vi "HFRR ADV v07 new software.vi"() -> ()   [LabVIEW 2025] (continued)
                frame 56 {
                  n3116 = local write "S 57"(w4150) -> ()
                }
                frame 57 {
                  n3117 = local write "S 58"(w4151) -> ()
                }
                frame 58 {
                  n3118 = local write "S 59"(w4152) -> ()
                }
                frame 59 {
                  n3119 = local write "S 60"(w4153) -> ()
                }
                frame 60 {
                  n3120 = local write "S 62"(w4154) -> ()
                }
                frame 61 {
                  n3121 = local write "S 63"(w4155) -> ()
                }
                frame 62 {
                  n3122 = local write "S 64"(w4156) -> ()
                }
                frame 63 {
                  n3123 = local write "S 65"(w4157) -> ()
                }
                frame 64 {
                  n3124 = local write "S 66"(w4158) -> ()
                }
                frame 65 {
                  n3125 = local write "S 67"(w4159) -> ()
                }
                frame 66 {
                  n3126 = local write "S 68"(w4160) -> ()
                }
                frame 67 {
                  n3127 = local write "S 69"(w4161) -> ()
                }
                frame 68 {
                  n3128 = local write "S 70"(w4162) -> ()
                }
                frame 69 {
                  n3129 = local write "S 71"(w4163) -> ()
                }
                frame 70 {
                  n3130 = local write "S 72"(w4164) -> ()
                }
                frame 71 {
                  n3131 = local write "S 73"(w4165) -> ()
                }
                frame 72 {
                  n3132 = local write "S 74"(w4166) -> ()
                }
                frame 73 {
                  n3133 = local write "S 75"(w4167) -> ()
                }
                frame 74 {
                  n3134 = local write "S 76"(w4168) -> ()
                }
                frame 75 {
                  n3135 = local write "S 77"(w4169) -> ()
                }
                frame 76 {
                  n3136 = local write "S 78"(w4170) -> ()
                }
                frame 77 {
                  n3137 = local write "S 79"(w4171) -> ()
                }
                frame 79 {
                  n3138 = property on="Sample Temperature ( °C )" class="XYGraph (strict)"("Y Scale.Name Label.Text"=w4172) -> ()  [unwired: 2 in, 2 out]
                }
                frame 80 {
                  n3139 = local write "S 81"(w4173) -> ()
                  n3140 = property on="Humidity ( %RH )" class="XYGraph (strict)"("Y Scale.Name Label.Text"=w4173) -> ()  [unwired: 2 in, 2 out]
                }
                frame 78 {
                  n3141 = property on="Air Temperature  ( °C )" class="XYGraph (strict)"("X Scale.Name Label.Text"=w4174) -> ()  [unwired: 2 in, 2 out]
                  n3142 = property on="Humidity ( %RH )" class="XYGraph (strict)"("X Scale.Name Label.Text"=w4174) -> ()  [unwired: 2 in, 2 out]
                  n3143 = property on="Sample Temperature ( °C )" class="XYGraph (strict)"("X Scale.Name Label.Text"=w4174) -> ()  [unwired: 2 in, 2 out]
                  n3144 = property on="Coefficient Of Friction" class="XYGraph (strict)"("X Scale.Name Label.Text"=w4174) -> ()  [unwired: 2 in, 2 out]
                }
                frame 81 {
                  n3145 = property on="Air Temperature  ( °C )" class="XYGraph (strict)"("Y Scale.Name Label.Text"=w4175) -> ()  [unwired: 2 in, 2 out]
                }
                frame 82 {
                  n3146 = local write "S 84"(w4176) -> ()
                }
                frame 83 {
                  n3147 = local write "S 85"(w4177) -> ()
                }
                frame 84 {
                  n3148 = local write "S 86"(w4178) -> ()
                }
                frame 85 {
                  n3149 = local write "S 87"(w4179) -> ()
                }
                frame 86 {
                  n3150 = local write "S 88"(w4180) -> ()
                }
                frame 87 {
                }
                frame 88 {
                  n3151 = local write "S 90"(w4182) -> ()
                }
                frame 89 {
                  n3152 = local write "S 91"(w4183) -> ()
                }
                frame 90 {
                  n3153 = local write "S 92"(w4184) -> ()
                }
                frame 91 {
                  n3154 = local write "S 93"(w4185) -> ()
                }
                frame 92 {
                  n3155 = local write "S 94"(w4186) -> ()
                }
                frame 93 {
                  n3156 = local write "S 95"(w4187) -> ()
                }
                frame 94 {
                  n3157 = local write "S 96"(w4188) -> ()
                }
                frame 95 {
                  n3158 = local write "S 97"(w4189) -> ()
                }
                frame 96 {
                  n3159 = local write "S 98"(w4190) -> ()
                }
                frame 97 {
                  n3160 = local write "S 99"(w4191) -> ()
                }
                frame 98 {
                  n3161 = local write "S 100"(w4192) -> ()
                }
                frame 99 {
                  n3162 = local write "S 101"(w4193) -> ()
                }
                frame 100 {
                  n3163 = local write "S 102"(w4194) -> ()
                }
                frame 101 {
                  n3164 = local write "S 103"(w4195) -> ()
                }
                frame 102 {
                  n3165 = local write "S 104"(w4196) -> ()
                }
                frame 103 {
                  n3166 = local write "S 105"(w4197) -> ()
                }
                frame 104 {
                  n3167 = local write "S 106"(w4198) -> ()
                }
                frame 105 {
                }
                frame 106 {
                  n3168 = property on="OK Button 17" class="Bool (strict)"("Boolean Text.Text"=w4199) -> ()  [unwired: 2 in, 2 out]
                }
                frame 107 {
                  n3169 = property on="OK Button 16" class="Bool (strict)"("Boolean Text.Text"=w4200) -> ()  [unwired: 2 in, 2 out]
                }
                frame 108 {
                  n3170 = property on="TITTLE" class="Str"("Caption.Text"=w4201) -> ()  [unwired: 2 in, 2 out]
                }
                frame 109 {
                  "String 30" <- w4202
                }
                frame 110 {
                  n3171 = property on="Test Date" class="Str"("Caption.Text"=w4203) -> ()  [unwired: 2 in, 2 out]
                  "String 31" <- w4203
                }
                frame 111 {
                  n3172 = property on="Sample ID" class="Str"("Caption.Text"=w4204) -> ()  [unwired: 2 in, 2 out]
                  "String 32" <- w4204
                }
                frame 112 {
                  n3173 = property on="Tested by" class="Str"("Caption.Text"=w4205) -> ()  [unwired: 2 in, 2 out]
                  "String 33" <- w4205
                }
                frame 113 {
                  n3174 = property on="System Configured Printers 2" class="Arr (strict)"("Caption.Text"=w4206) -> ()  [unwired: 2 in, 2 out]
                }
                frame 114 {
                  n3175 = property on="Selected Printer" class="Str"("Caption.Text"=w4207) -> ()  [unwired: 2 in, 2 out]
                }
                frame 115 {
                  n3176 = property on="Select Printer 3" class="DigNum (strict)"("Caption.Text"=w4208) -> ()  [unwired: 2 in, 2 out]
                }
                frame 116 {
                  n3177 = property on="Print" class="Bool (strict)"("Boolean Text.Text"=w4209) -> ()  [unwired: 2 in, 2 out]
                }
                frame 117 {
                  "String 41" <- w4210
                }
                frame 118 {
                  n3178 = property on="tested by" class="Str"("Caption.Text"=w4211) -> ()  [unwired: 2 in, 2 out]
                }
                frame 119 {
                }
                frame 120 {
                  n3179 = property on="Export" class="Bool (strict)"("Boolean Text.Text"=w4212) -> ()  [unwired: 2 in, 2 out]
                }
                frame 121 {
                  n3180 = property on="TEMP INTERCEPT:" class="DigNum (strict)"("Caption.Text"=w4213) -> ()  [unwired: 2 in, 2 out]
                }
                frame 122 {
                  n3181 = property on="AIR TEMP INTERCEPT:" class="DigNum (strict)"("Caption.Text"=w4214) -> ()  [unwired: 2 in, 2 out]
                }
                frame 123 {
                  n3182 = property on="Select File Type" class="Enum (strict)"("Caption.Text"=w4215) -> ()  [unwired: 2 in, 2 out]
                }
                frame 124 {
                  n3183 = property on="s.NO" class="Str"("Caption.Text"=w4216) -> ()  [unwired: 2 in, 2 out]
                  "String 45" <- w4216
                }
                frame 125 {
                  n3184 = property on="trip1 8" class="Bool (strict)"("Boolean Text.Text"=w4217) -> ()  [unwired: 2 in, 2 out]
                }
                frame 126, Default {
                }
              }
            }
          }
          frame #1 {
            w4225 = TRUE ("Visible")
            n3185 = local read "S 91"() -> (w4242:string)
            n3186 = local read "S 90"() -> (w4241:string)
            n3187 = local read "S 88"() -> (w4240:string)
            n3188 = property on="File Path" class="Path"("Caption.Text"=w4241) -> ()  [unwired: 2 in, 2 out]
            n3189 = property on="SrvM CP" class="Bool (strict)"("Boolean Text.Text"=w4240) -> ()  [unwired: 2 in, 2 out]
            n3190 = local read "S 71"() -> (w4235:string)
            n3191 = local read "S 86"() -> (w4237:string)
            n3192 = local read "S 85"() -> (w4238:string)
            n3193 = local read "S 87"() -> (w4236:string)
            n3194 = local read "S 84"() -> (w4239:string)
            n3195 = local read "S 103"() -> (w4224:string)
            n3196 = local read "S 104"() -> (w4223:string)
            n3197 = property on="ENTER THE NEW PASSWORD" class="Str"("Caption.Text"=w4236) -> ()  [unwired: 2 in, 2 out]
            n3198 = property on="Password" class="Str"("Caption.Text"=w4238) -> ()  [unwired: 2 in, 2 out]
            n3199 = property on="ENTER CURRENT PASSWORD" class="Str"("Caption.Text"=w4237) -> ()  [unwired: 2 in, 2 out]
            n3200 = property on="EDIT" class="Bool (strict)"("Boolean Text.Text"=w4235) -> ()  [unwired: 2 in, 2 out]
            n3201 = property on="SAVE" class="Bool (strict)"("Boolean Text.Text"=w4239) -> ()  [unwired: 2 in, 2 out]
            n3202 = Build Array(w4224, w4223) -> (w4222:string[])
            n3203 = property on="Heater Button" class="Bool (strict)"("Strings [4]"=w4222) -> ()  [unwired: 2 in, 2 out]
            n3204 = property on="CH-HUMIDITY WET" class="DigNum (strict)"("Caption.Size to Text?"=w4225) -> ()  [unwired: 2 in, 2 out]
            n3205 = property on="CH-HUMIDITY DRY" class="DigNum (strict)"("Caption.Size to Text?"=w4225) -> ()  [unwired: 2 in, 2 out]
            n3206 = property on="CH-POWER -" class="DigNum (strict)"("Caption.Size to Text?"=w4225) -> ()  [unwired: 2 in, 2 out]
            n3207 = property on="CH-HEATER" class="DigNum (strict)"("Caption.Size to Text?"=w4225) -> ()  [unwired: 2 in, 2 out]
            n3208 = property on="CH-POWER +" class="DigNum (strict)"("Caption.Size to Text?"=w4225) -> ()  [unwired: 2 in, 2 out]
            n3209 = local read "S 92"() -> (w4234:string)
            n3210 = local read "S 93"() -> (w4233:string)
            n3211 = local read "S 105"() -> (w4220:string)
            n3212 = local read "S 106"() -> (w4219:string)
            n3213 = Build Array(w4234, w4233) -> ()  [unwired: 1 out]
            n3214 = Build Array(w4220, w4219) -> (w4221:string[])
            n3215 = local read "S 95"() -> (w4231:string)
            n3216 = local read "S 94"() -> (w4232:string)
            n3217 = local read "bs"() -> (w4247:string)
            n3218 = local read "as"() -> (w4248:string)
            n3219 = property on="Humidity" class="Bool (strict)"("Strings [4]"=w4221) -> ()  [unwired: 2 in, 2 out]
            n3220 = Concatenate Strings(w4247, "\r", w4248) -> ()  [unwired: 1 out]
            n3221 = property on="STROKE GAIN :" class="DigNum (strict)"("Caption.Text"=w4231) -> ()  [unwired: 2 in, 2 out]
            n3222 = property on="DISPLACEMENT :" class="DigNum (strict)"("Caption.Text"=w4232) -> ()  [unwired: 2 in, 2 out]
            n3223 = property on="Rh After" class="DigNum (strict)"("Caption.Size to Text?"=TRUE ("Caption.Size to Text")) -> ()  [unwired: 2 in, 2 out]
            n3224 = local read "S 48"() -> (w4271:string)
            n3225 = local read "S 50"() -> (w4269:string)
            n3226 = local read "S 51"() -> (w4268:string)
            n3227 = local read "S 49"() -> (w4270:string)
            n3228 = local read "S 52"() -> (w4267:string)
            n3229 = local read "as"() -> (w4252:string)
            n3230 = local read "bs"() -> (w4253:string)
            n3231 = local read "S 56"() -> (w4266:string)
            n3232 = local read "S 57"() -> (w4265:string)
            n3233 = local read "S 58"() -> (w4264:string)
            n3234 = local read "S 59"() -> (w4263:string)
            n3235 = property on="OPEN" class="Bool (strict)"("Boolean Text.Text"=w4267) -> ()  [unwired: 2 in, 2 out]
            n3236 = property on="OPEN 1" class="Bool (strict)"("Boolean Text.Text"=w4271) -> ()  [unwired: 2 in, 2 out]
            n3237 = property on="OPEN 2" class="Bool (strict)"("Boolean Text.Text"=w4270) -> ()  [unwired: 2 in, 2 out]
            n3238 = property on="OPEN 3" class="Bool (strict)"("Boolean Text.Text"=w4269) -> ()  [unwired: 2 in, 2 out]
            n3239 = property on="OPEN 4" class="Bool (strict)"("Boolean Text.Text"=w4268) -> ()  [unwired: 2 in, 2 out]
            n3240 = Concatenate Strings(w4253, "\r", w4252) -> ()  [unwired: 1 out]
            n3241 = local read "S 102"() -> (w4226:string)
            n3242 = property on="КОФ1" class="DigNum (strict)"("Caption.Text"=w4266) -> ()  [unwired: 2 in, 2 out]
            n3243 = local read "S 98"() -> (w4230:string)
            n3244 = local read "S 99"() -> (w4229:string)
            n3245 = local read "S 100"() -> (w4228:string)
            n3246 = local read "S 101"() -> (w4227:string)
            n3247 = property on="КОФ2" class="DigNum (strict)"("Caption.Text"=w4265) -> ()  [unwired: 2 in, 2 out]
            n3248 = property on="КОФ3" class="DigNum (strict)"("Caption.Text"=w4264) -> ()  [unwired: 2 in, 2 out]
            n3249 = property on="КОФ4" class="DigNum (strict)"("Caption.Text"=w4263) -> ()  [unwired: 2 in, 2 out]
            n3250 = local read "bs"() -> (w4251:string)
            n3251 = local read "as"() -> (w4250:string)
            n3252 = property on="CH-POWER +" class="DigNum (strict)"("Caption.Text"=w4230) -> ()  [unwired: 2 in, 2 out]
            n3253 = property on="CH-POWER -" class="DigNum (strict)"("Caption.Text"=w4229) -> ()  [unwired: 2 in, 2 out]
            n3254 = property on="CH-HEATER" class="DigNum (strict)"("Caption.Text"=w4228) -> ()  [unwired: 2 in, 2 out]
            n3255 = property on="CH-HUMIDITY DRY" class="DigNum (strict)"("Caption.Text"=w4227) -> ()  [unwired: 2 in, 2 out]
            n3256 = property on="CH-HUMIDITY WET" class="DigNum (strict)"("Caption.Text"=w4226) -> ()  [unwired: 2 in, 2 out]
            n3257 = local read "S 60"() -> (w4262:string)
            n3258 = local read "S 54"() -> (w4272:string)
            n3259 = Concatenate Strings(w4251, "\r", w4250) -> ()  [unwired: 1 out]
            n3260 = Concatenate Strings(w4272, w4262) -> ()  [unwired: 1 out]
            n3261 = local read "S 77"() -> (→"String 43":string)
            n3262 = local read "S 76"() -> (w4245:string)
            n3263 = local read "S 78"() -> (w4244:string)
            n3264 = local read "S 71"() -> (w4256:string)
            n3265 = local read "S 66"() -> (w4261:string)
            n3266 = local read "S 67"() -> (w4260:string)
            n3267 = local read "S 68"() -> (w4259:string)
            n3268 = local read "S 69"() -> (w4258:string)
            n3269 = local read "S 70"() -> (w4257:string)
            n3270 = property on="AIR TEMP" class="DigNum (strict)"("Caption.Text"=w4244) -> ()  [unwired: 2 in, 2 out]
            n3271 = property on="Set Strk" class="DigNum (strict)"("Caption.Text"=w4245) -> ()  [unwired: 2 in, 2 out]
            n3272 = property on="FRIC. FORCE :" class="DigNum (strict)"("Caption.Text"=w4261) -> ()  [unwired: 2 in, 2 out]
            n3273 = property on="TEMPERATURE :" class="DigNum (strict)"("Caption.Text"=w4260) -> ()  [unwired: 2 in, 2 out]
            n3274 = property on="SPEED OUT:" class="DigNum (strict)"("Caption.Text"=w4259) -> ()  [unwired: 2 in, 2 out]
            n3275 = property on="AIR TEMPERATURE :" class="DigNum (strict)"("Caption.Text"=w4258) -> ()  [unwired: 2 in, 2 out]
            n3276 = property on="HUMIDITY:" class="DigNum (strict)"("Caption.Text"=w4257) -> ()  [unwired: 2 in, 2 out]
            n3277 = property on="EDIT" class="Bool (strict)"("Boolean Text.Text"=w4256) -> ()  [unwired: 2 in, 2 out]
            n3278 = local read "S 79"() -> (w4243:string)
          }
          frame #2 {
          }
        }
        n3279 = local write "Lan flag"(10.0 ("Lan flag")) -> ()
      }
      frame Enabled {
      }
    }
    n3280 = Wait (ms)(milliseconds to wait=u32 2000) -> ()  [unwired: 1 out]
    n3281 = local read "Quit"() -> (w4046:bool)
  }
  n3282 = disable-structure shown="Disabled" {
    frame Disabled {
      n3283 = while {
        tunnel: [w4274] -> _
        i -> [w4274]
        stop <- w4273 continue-if-true
        n3284 = Wait (ms)(milliseconds to wait=u32 50) -> ()  [unwired: 1 out]
        n3285 = stacked-sequence {
          frame #0 {
            # "Controls Text color"
            # "Controls BG color"
            n3286 = property on="FILE" class="Str"("Text.Text Colors:Text Color"="SC  Text") -> ()  [unwired: 2 in, 2 out]
            n3287 = property on="Fuel Discription :" class="Str"("Text.Text Colors:Text Color"="SC  Text") -> ()  [unwired: 2 in, 2 out]
            n3288 = property on="tested by" class="Str"("Text.Text Colors:Text Color"="SC  Text") -> ()  [unwired: 2 in, 2 out]
            n3289 = property on="Remarks :" class="Str"("Text.Text Colors:Text Color"="SC  Text") -> ()  [unwired: 2 in, 2 out]
            n3290 = property class="DigNum (strict)"("Numeric Text.Text Colors:BG Color"="NC BG") -> ()  [unwired: 2 in, 2 out]
            n3291 = property class="DigNum (strict)"("Numeric Text.Text Colors:BG Color"="NC BG") -> ()  [unwired: 2 in, 2 out]
            n3292 = property class="DigNum (strict)"("Numeric Text.Text Colors:BG Color"="NC BG") -> ()  [unwired: 2 in, 2 out]
            n3293 = property class="DigNum (strict)"("Numeric Text.Text Colors:BG Color"="NC BG") -> ()  [unwired: 2 in, 2 out]
            n3294 = property class="DigNum (strict)"("Numeric Text.Text Colors:BG Color"="NC BG") -> ()  [unwired: 2 in, 2 out]
            n3295 = property class="DigNum (strict)"("Numeric Text.Text Colors:BG Color"="NC BG") -> ()  [unwired: 2 in, 2 out]
            n3296 = property class="DigNum (strict)"("Numeric Text.Text Colors:BG Color"="NC BG") -> ()  [unwired: 2 in, 2 out]
            n3297 = property class="DigNum (strict)"("Numeric Text.Text Colors:BG Color"="NC BG") -> ()  [unwired: 2 in, 2 out]
            n3298 = property class="DigNum (strict)"("Numeric Text.Text Colors:BG Color"="NC BG") -> ()  [unwired: 2 in, 2 out]
            n3299 = property class="DigNum (strict)"("Numeric Text.Text Colors:BG Color"="NC BG") -> ()  [unwired: 2 in, 2 out]
            n3300 = property class="DigNum (strict)"("Numeric Text.Text Colors:BG Color"="NC BG") -> ()  [unwired: 2 in, 2 out]
            n3301 = property class="DigNum (strict)"("Numeric Text.Text Colors:BG Color"="NC BG") -> ()  [unwired: 2 in, 2 out]
            n3302 = property on="FILE" class="Str"("Text.Text Colors:BG Color"="SC BG 3") -> ()  [unwired: 2 in, 2 out]
            n3303 = property on="Fuel Discription :" class="Str"("Text.Text Colors:BG Color"="SC BG 3") -> ()  [unwired: 2 in, 2 out]
            n3304 = property on="tested by" class="Str"("Text.Text Colors:BG Color"="SC BG 3") -> ()  [unwired: 2 in, 2 out]
            n3305 = property on="Remarks :" class="Str"("Text.Text Colors:BG Color"="SC BG 3") -> ()  [unwired: 2 in, 2 out]
            n3306 = property class="DigNum (strict)"("Numeric Text.Text Colors:Text Color"="NC Text") -> ()  [unwired: 2 in, 2 out]
            n3307 = property class="DigNum (strict)"("Numeric Text.Text Colors:Text Color"="NC Text") -> ()  [unwired: 2 in, 2 out]
            n3308 = property class="DigNum (strict)"("Numeric Text.Text Colors:Text Color"="NC Text") -> ()  [unwired: 2 in, 2 out]
            n3309 = property class="DigNum (strict)"("Numeric Text.Text Colors:Text Color"="NC Text") -> ()  [unwired: 2 in, 2 out]
            n3310 = property class="DigNum (strict)"("Numeric Text.Text Colors:Text Color"="NC Text") -> ()  [unwired: 2 in, 2 out]
            n3311 = property class="DigNum (strict)"("Numeric Text.Text Colors:Text Color"="NC Text") -> ()  [unwired: 2 in, 2 out]
            n3312 = property class="DigNum (strict)"("Numeric Text.Text Colors:Text Color"="NC Text") -> ()  [unwired: 2 in, 2 out]
            n3313 = property class="DigNum (strict)"("Numeric Text.Text Colors:Text Color"="NC Text") -> ()  [unwired: 2 in, 2 out]
            n3314 = property class="DigNum (strict)"("Numeric Text.Text Colors:Text Color"="NC Text") -> ()  [unwired: 2 in, 2 out]
            n3315 = property class="DigNum (strict)"("Numeric Text.Text Colors:Text Color"="NC Text") -> ()  [unwired: 2 in, 2 out]
            n3316 = property class="DigNum (strict)"("Numeric Text.Text Colors:Text Color"="NC Text") -> ()  [unwired: 2 in, 2 out]
            n3317 = property class="DigNum (strict)"("Numeric Text.Text Colors:Text Color"="NC Text") -> ()  [unwired: 2 in, 2 out]
            n3318 = property class="DigNum (strict)"("Numeric Text.Text Colors:Text Color"="NI Text  2") -> ()  [unwired: 2 in, 2 out]
            n3319 = property class="DigNum (strict)"("Numeric Text.Text Colors:Text Color"="NI Text  2") -> ()  [unwired: 2 in, 2 out]
            n3320 = property class="DigNum (strict)"("Numeric Text.Text Colors:Text Color"="NI Text  2") -> ()  [unwired: 2 in, 2 out]
            n3321 = property class="DigNum (strict)"("Numeric Text.Text Colors:Text Color"="NI Text  2") -> ()  [unwired: 2 in, 2 out]
            n3322 = property class="DigNum (strict)"("Numeric Text.Text Colors:Text Color"="NI Text  2") -> ()  [unwired: 2 in, 2 out]
            n3323 = property class="DigNum (strict)"("Numeric Text.Text Colors:Text Color"="NI Text  2") -> ()  [unwired: 2 in, 2 out]
            n3324 = property class="DigNum (strict)"("Numeric Text.Text Colors:Text Color"="NI Text  2") -> ()  [unwired: 2 in, 2 out]
            n3325 = property class="DigNum (strict)"("Numeric Text.Text Colors:Text Color"="NI Text  2") -> ()  [unwired: 2 in, 2 out]
            n3326 = property class="DigNum (strict)"("Numeric Text.Text Colors:Text Color"="NI Text  2") -> ()  [unwired: 2 in, 2 out]
            n3327 = property class="DigNum (strict)"("Numeric Text.Text Colors:Text Color"="NI Text  2") -> ()  [unwired: 2 in, 2 out]
            n3328 = property class="DigNum (strict)"("Numeric Text.Text Colors:Text Color"="NI Text  2") -> ()  [unwired: 2 in, 2 out]
            n3329 = property class="DigNum (strict)"("Numeric Text.Text Colors:Text Color"="NI Text  2") -> ()  [unwired: 2 in, 2 out]
            n3330 = property class="DigNum (strict)"("Numeric Text.Text Colors:Text Color"="NI Text  2") -> ()  [unwired: 2 in, 2 out]
            n3331 = property class="DigNum (strict)"("Numeric Text.Text Colors:Text Color"="NI Text  2") -> ()  [unwired: 2 in, 2 out]
            n3332 = property class="DigNum (strict)"("Numeric Text.Text Colors:Text Color"="NI Text  2") -> ()  [unwired: 2 in, 2 out]
            n3333 = property on="Coefficient Of Friction" class="XYGraph (strict)"("Plot Area:Colors:FG Color"="GFG  2", "Plot Area:Colors:BG Color"="GBG   2") -> ()  [unwired: 2 in, 2 out]
            n3334 = property on="Humidity ( %RH )" class="XYGraph (strict)"("Plot Area:Colors:FG Color"="GFG  2", "Plot Area:Colors:BG Color"="GBG   2") -> ()  [unwired: 2 in, 2 out]
            n3335 = property on="Air Temperature  ( °C )" class="XYGraph (strict)"("Plot Area:Colors:FG Color"="GFG  2", "Plot Area:Colors:BG Color"="GBG   2") -> ()  [unwired: 2 in, 2 out]
            n3336 = property on="Sample Temperature ( °C )" class="XYGraph (strict)"("Plot Area:Colors:FG Color"="GFG  2", "Plot Area:Colors:BG Color"="GBG   2") -> ()  [unwired: 2 in, 2 out]
            n3337 = property class="DigNum (strict)"("Numeric Text.Text Colors:BG Color"="NI BG 2") -> ()  [unwired: 2 in, 2 out]
            n3338 = property class="DigNum (strict)"("Numeric Text.Text Colors:BG Color"="NI BG 2") -> ()  [unwired: 2 in, 2 out]
            n3339 = property class="DigNum (strict)"("Numeric Text.Text Colors:BG Color"="NI BG 2") -> ()  [unwired: 2 in, 2 out]
            n3340 = property class="DigNum (strict)"("Numeric Text.Text Colors:BG Color"="NI BG 2") -> ()  [unwired: 2 in, 2 out]
            n3341 = property class="DigNum (strict)"("Numeric Text.Text Colors:BG Color"="NI BG 2") -> ()  [unwired: 2 in, 2 out]
            n3342 = property class="DigNum (strict)"("Numeric Text.Text Colors:BG Color"="NI BG 2") -> ()  [unwired: 2 in, 2 out]
            n3343 = property class="DigNum (strict)"("Numeric Text.Text Colors:BG Color"="NI BG 2") -> ()  [unwired: 2 in, 2 out]
            n3344 = property class="DigNum (strict)"("Numeric Text.Text Colors:BG Color"="NI BG 2") -> ()  [unwired: 2 in, 2 out]
            n3345 = property class="DigNum (strict)"("Numeric Text.Text Colors:BG Color"="NI BG 2") -> ()  [unwired: 2 in, 2 out]
            n3346 = property class="DigNum (strict)"("Numeric Text.Text Colors:BG Color"="NI BG 2") -> ()  [unwired: 2 in, 2 out]
            n3347 = property class="DigNum (strict)"("Numeric Text.Text Colors:BG Color"="NI BG 2") -> ()  [unwired: 2 in, 2 out]
            n3348 = property class="DigNum (strict)"("Numeric Text.Text Colors:BG Color"="NI BG 2") -> ()  [unwired: 2 in, 2 out]
            n3349 = property class="DigNum (strict)"("Numeric Text.Text Colors:BG Color"="NI BG 2") -> ()  [unwired: 2 in, 2 out]
            n3350 = property class="DigNum (strict)"("Numeric Text.Text Colors:BG Color"="NI BG 2") -> ()  [unwired: 2 in, 2 out]
            n3351 = property class="DigNum (strict)"("Numeric Text.Text Colors:BG Color"="NI BG 2") -> ()  [unwired: 2 in, 2 out]
            n3352 = property class="Bool"("Colors [4]"="Boolean BC T & BG") -> ()  [unwired: 2 in, 2 out]
            n3353 = property on="Save & Continue" class="Bool (strict)"("Colors [4]"="Boolean BC T & BG") -> ()  [unwired: 2 in, 2 out]
            n3354 = property on="Heater Button" class="Bool (strict)"("Colors [4]"="Boolean BC T & BG") -> ()  [unwired: 2 in, 2 out]
            n3355 = property class="Bool"("Colors [4]"="Boolean BC T & BG") -> ()  [unwired: 2 in, 2 out]
            n3356 = property on="Humidity" class="Bool (strict)"("Colors [4]"="Boolean BC T & BG") -> ()  [unwired: 2 in, 2 out]
            n3357 = property class="Bool (strict)"("Colors [4]"="Boolean BC T & BG") -> ()  [unwired: 2 in, 2 out]
            n3358 = property on="RUN" class="Bool (strict)"("Colors [4]"="Boolean BC T & BG") -> ()  [unwired: 2 in, 2 out]
            n3359 = property on="trip1 8" class="Bool (strict)"("Colors [4]"="Boolean BC T & BG") -> ()  [unwired: 2 in, 2 out]
            n3360 = property class="Bool"("Colors [4]"="Boolean BC T & BG") -> ()  [unwired: 2 in, 2 out]
            n3361 = property class="Bool (strict)"("Colors [4]"="Boolean BC T & BG") -> ()  [unwired: 2 in, 2 out]
            n3362 = property on="OPEN 1" class="Bool (strict)"("Colors [4]"="Boolean BC T & BG 2") -> ()  [unwired: 2 in, 2 out]
            n3363 = property on="OPEN 2" class="Bool (strict)"("Colors [4]"="Boolean BC T & BG 2") -> ()  [unwired: 2 in, 2 out]
            n3364 = property on="OPEN 3" class="Bool (strict)"("Colors [4]"="Boolean BC T & BG 2") -> ()  [unwired: 2 in, 2 out]
            n3365 = property on="OPEN 4" class="Bool (strict)"("Colors [4]"="Boolean BC T & BG 2") -> ()  [unwired: 2 in, 2 out]
            n3366 = property on="OPEN" class="Bool (strict)"("Colors [4]"="Boolean BC T & BG 2") -> ()  [unwired: 2 in, 2 out]
            n3367 = property on="rstv2" class="Bool"("Colors [4]"="Boolean BC T & BG 2") -> ()  [unwired: 2 in, 2 out]
            n3368 = property on="RST CP" class="Bool"("Colors [4]"="Boolean BC T & BG 2") -> ()  [unwired: 2 in, 2 out]
            n3369 = property on="RSTV1 3" class="Bool"("Colors [4]"="Boolean BC T & BG 2") -> ()  [unwired: 2 in, 2 out]
            n3370 = property on="RSTV1 2" class="Bool"("Colors [4]"="Boolean BC T & BG 2") -> ()  [unwired: 2 in, 2 out]
          }
          frame #1 {
          }
        }
        n3371 = local read "Quit"() -> (w4273:bool)
      }
    }
    frame Enabled {
    }
  }
  n3372 = while {
    shift-right: [w4291] -> _
    shift-left: _ -> [w4292]
    shift-right: [w4289] -> _
    shift-left: T16 {"Read Heave and Surge"="", "Bytes at Heave Port"=0.0, "Heave and Surge COM Port:"="COM9", "Com Port 2"="COM7", "Residual Due"="", "Heave COM Status 2"=TRUE, "Heave COM Status"=TRUE, "Port 2"=TRUE, "Sway PPR"=6400.0, "Surge PPR"=6400.0, "Heave PPR"=6400.0, "Sway Pitch"=2.0, "Surge Pitch"=3.0, "Heave Pitch"=4.0, "Sway Pulses/mm"=320.0, "Surge Pulses/mm"=1600.0, "Heave Pulses/mm"=1600.0, "inner loop"=0.0, "Read Heave and Surge 2"="", "String 36"="", "Write S"=FALSE, "WriteCC1"=[""], "Heave COM Loop"=0, "LastCom"="", "EXIT"=FALSE, "Error Heave"={"status"=TRUE, "code"=-1073807343, "source"=""}} -> [w4288]
    shift-right: [w4286] -> _
    shift-left: enum16{"init", "MAIN", "Panel Close"}."init" -> [w4287]
    stop <- w4290 stop-if-true
    n3373 = case shown="\"MAIN\"" w4287 {
      tunnel: w4292 -> [w4306 w4321 w4391 w4393]
      tunnel: [w4300 w4339 w4391 w4393] -> w4291
      tunnel: [_ _ TRUE _] -> w4290
      tunnel: [w4296 w4336 w4389 w4392] -> w4289
      tunnel: w4288 -> [w4303 w4320 w4389 w4392]
      tunnel: [enum16{"init", "MAIN", "Panel Close"}."MAIN" w4314 _ _] -> w4286
      frame "init" {
        n3374 = Bundle By Name(cluster=w4303, "Heave and Surge COM Port:"="C3 :") -> (w4302:T16)
        n3375 = call "Instrument fgv.vi"("Enum"=T28."INIT", "error in (no error) 2"=w4306, "INPUT"=w4302) -> ("error"=w4304:errorcluster, "output"=w4299:T16)  [unwired: 6 in, 1 out]
        n3376 = case shown="No Error" w4304 {
          selector: w4304 -> [w4308 _]
          tunnel: [w4308 w4312] -> w4300
          tunnel: w4299 -> [w4307 w4310]
          tunnel: [w4307 w4309] -> w4297
          frame No Error {
          }
          frame Error {
            n3377 = call "Instrument fgv.vi"("Enum"=T28."ERROR INIT", "INPUT"=w4310) -> ("error"=w4313:errorcluster, "output"=w4309:T16)  [unwired: 7 in, 1 out]
            n3378 = call <vilib>:"Clear Errors.vi"("error in (no error)"=w4313) -> ("error out"=w4312:errorcluster)  [unwired: 5 in, 1 out]
          }
        }
        n3379 = local read "LastCom"() -> (w4295:string)
        n3380 = Unbundle By Name(w4297) -> ("Heave COM Status 2"=→"COM Status" →"Instrument Status":bool, "Error Heave"=→"Error":errorcluster)  [unwired: 1 out]
        n3381 = Bundle By Name(cluster=w4297, "LastCom"=w4295) -> (w4296:T16)
      }
      frame "MAIN" {
        n3382 = Unbundle By Name(w4320) -> ("Com Port 2"=w4341:refnum<visa-resource-name>)
        n3383 = local write "Com Port 4"(w4341) -> ()
        n3384 = local read "C3 :"() -> (w4318:refnum<visa-resource-name>)
        n3385 = Divide(x="Heave PPR", y="Heave Pitch") -> (x/y=→"Heave Pulses/mm":dbl)
        n3386 = Bundle By Name(cluster=w4320, "Heave and Surge COM Port:"=w4318) -> (w4319:T16)
        n3387 = Equal?(x=w4341, y=w4318) -> (x = y?=w4340:bool)
        n3388 = Divide(x="Sway PPR", y="Sway Pitch") -> (x/y=→"Sway Pulses/mm":dbl)
        n3389 = case shown="False" w4340 {
          tunnel: [w4345 w4362] -> w4339
          tunnel: w4321 -> [w4346 w4368]
          tunnel: w4319 -> [w4344 w4366]
          tunnel: [w4343 w4361] -> w4336
          frame False {
            n3390 = call <vilib>:"Clear Errors.vi"("error in (no error)"=w4346) -> ("error out"=w4342:errorcluster)  [unwired: 5 in, 1 out]
            n3391 = call "Instrument fgv.vi"("Enum"=T28."ERROR INIT", "error in (no error) 2"=w4342, "INPUT"=w4344) -> ("error"=w4348:errorcluster, "output"=w4343:T16)  [unwired: 6 in, 1 out]
            n3392 = call <vilib>:"Clear Errors.vi"("error in (no error)"=w4348) -> ("error out"=w4345:errorcluster)  [unwired: 5 in, 1 out]
          }
          frame True {
            n3393 = call "Instrument fgv.vi"("Enum"=T28."READ", "error in (no error) 2"=w4368, "INPUT"=w4366) -> ("error"=w4367:errorcluster, "output"=w4358:T16)  [unwired: 6 in, 1 out]
            n3394 = Bundle By Name(cluster=w4358, "String 36"="String 11") -> (w4357:T16)
            n3395 = case shown="True" "Write S" {
              selector: "Write S" -> [_ w4388]
              tunnel: w4367 -> [w4381 w4387]
              tunnel: [w4381 w4386] -> w4354
              tunnel: w4357 -> [w4380 w4383]
              tunnel: [w4380 w4382] -> w4353
              frame False {
              }
              frame True {
                n3396 = Not(x=w4388) -> (.not. x?=w4384:bool)
                n3397 = local write "Write S"(w4384) -> ()
                n3398 = call "Instrument fgv.vi"("Enum"=T28."MANUAL WRITE", "error in (no error) 2"=w4387, "INPUT"=w4383) -> ("error"=w4386:errorcluster, "output"=w4382:T16)  [unwired: 6 in, 1 out]
              }
            }
            n3399 = Array Size(array="WriteHumidity") -> (size(s)=w4351:i32)
            n3400 = Greater Than 0?(x=w4351) -> (x > 0?=w4349:bool)
            n3401 = call "Instrument fgv.vi"("Enum"=T28."WRITE", "error in (no error) 2"=w4354, "WriteCC1"="WriteHumidity", "INPUT"=w4353) -> ("error"=w4364:errorcluster, "WriteCC1 2"=w4352:string[], "output"=w4363:T16)  [unwired: 5 in]
            n3402 = case shown="True" w4349 {
              tunnel: w4352 -> [_ w4370]
              frame False {
              }
              frame True {
                n3403 = local write "WriteHumidity"(w4370) -> ()
              }
            }
            n3404 = case shown="Error" w4364 {
              selector: w4364 -> [w4371 w4374]
              tunnel: w4363 -> [w4372 w4379]
              tunnel: [w4372 w4378] -> w4361
              tunnel: [w4371 w4376] -> w4362
              frame No Error {
              }
              frame Error {
                n3405 = call <vilib>:"Clear Errors.vi"("error in (no error)"=w4374) -> ("error out"=w4373:errorcluster)  [unwired: 5 in, 1 out]
                n3406 = call "Instrument fgv.vi"("Enum"=T28."ERROR INIT", "error in (no error) 2"=w4373, "INPUT"=w4379) -> ("error"=w4377:errorcluster, "output"=w4378:T16)  [unwired: 6 in, 1 out]
                n3407 = call <vilib>:"Clear Errors.vi"("error in (no error)"=w4377) -> ("error out"=w4376:errorcluster)  [unwired: 5 in, 1 out]
              }
            }
            n3408 = Unbundle By Name(w4361) -> ("LastCom"=→"LastCom":string, "Read Heave and Surge"=→"Read Humidity":string)
          }
        }
        n3409 = Divide(x="Surge PPR", y="Surge Pitch") -> (x/y=→"Surge Pulses/mm":dbl)
        n3410 = Unbundle By Name(w4336) -> ("Heave COM Status 2"=w4338:bool, "Heave COM Status"=w4337:bool, "Error Heave"=w4334:errorcluster, "Bytes at Heave Port"=→"Bytes at Humidity Port":dbl)
        n3411 = Unbundle By Name(w4334) -> ("status"=→"Humidity Port":bool)
        n3412 = Not(x=w4337) -> (.not. x?=w4322:bool)
        n3413 = local write "Error"(w4334) -> ()
        n3414 = Not(x=w4338) -> (.not. x?=w4323:bool)
        n3415 = local write "Instrument Status"(w4322) -> ()
        n3416 = local write "COM Status"(w4323) -> ()
        n3417 = local read "Quit"() -> (w4315:bool)
        n3418 = Select(t=enum16{"init", "MAIN", "Panel Close"}."Panel Close", s=w4315, f=enum16{"init", "MAIN", "Panel Close"}."MAIN") -> (s? t:f=w4314:enum16{"init", "MAIN", "Panel Close"})
      }
      frame "Panel Close" {
      }
      frame Default {
      }
    }
  }
  n3419 = while {
    stop <- w4419 stop-if-true
    n3420 = local read "Read Humidity"() -> (w4400:string)
    n3421 = call <vilib>:"High Resolution Polling Wait.vi"("seconds to wait"=0.1) -> ()  [unwired: 10 in, 1 out]
    n3422 = Spreadsheet String To Array(delimiter (Tab)=",", format string="", spreadsheet string=w4400, array type (2D Dbl)=string[] []) -> (array=w4414:string[])
    n3423 = for {
      tunnel: w4414 -> [w4424] mode=indexing
      tunnel: string[] ["STATE;", "SET;", "RH;", "T;", "AMB_RH;", "AMB_T;", "PUMP;", "FAN_IN;", "FAN_OUT;", "DEHUM;", "CURRENT;", "STALL;"] -> [w4423] mode=indexing
      tunnel: [w4422] -> w4413 mode=indexing
      n3424 = Match Pattern(string=w4424, regular expression=w4423) -> (after substring=w4422:string)  [unwired: 1 in, 3 out]
    }
    n3425 = Index Array(array=w4413) -> (element #1=→"STATE :":string, element #2=→"SET :":string, element #3=w4402:string, element #4=→"T :":string, element #5=w4399:string, element #6=→"AMB_T :":string, element #7=→"PUMP :":string, element #8=→"FAN_IN :":string, element #9=→"FAN_OUT :":string, element #10=→"DEHUM :":string, element #11=→"CURRENT :":string, element #12=→"STALL :":string)  [unwired: 12 in]
    "RH :" <- w4402
    "AMB_RH :" <- w4399
    n3426 = Fract/Exp String To Number(string=w4402) -> (number=w4394:dbl)  [unwired: 3 in, 1 out]
    n3427 = Fract/Exp String To Number(string=w4399) -> (number=w4398:dbl)  [unwired: 3 in, 1 out]
    n3428 = local write "Ambient Humidity :"(w4398) -> ()
    n3429 = Equal?(x=w4394, y=0.0) -> (x = y?=w4396:bool)
    n3430 = case shown="True" w4396 {
      tunnel: [w4420 w4421] -> w4395
      tunnel: w4394 -> [w4420 _]
      frame False {
        (unwired) 0.0
        "Humidity temp" <- w4420
      }
      frame True {
        n3431 = local read "Humidity temp"() -> (w4421:dbl)
      }
    }
    "RH Numeric:" <- w4395
    n3432 = local read "Quit"() -> (w4419:bool)
  }
  n3433 = disable-structure shown="Disabled" {
    frame Disabled {
      n3434 = while {
        tunnel: [w4658] -> _
        i -> [w4658]
        stop <- w4655 stop-if-true
        n3435 = local read "powstat"() -> (w4656:bool)
        n3436 = case shown="True" w4656 {
          frame False {
          }
          frame True {
            n3437 = local read "RUN"() -> (w4659:bool)
            n3438 = case shown="True" w4659 {
              frame False {
                w4689 = 65.0 ("y")
                n3439 = local read "Set Hz"() -> (w4717:dbl)
                n3440 = local read "NORMAL LOAD"() -> (w4718:dbl)
                n3441 = Multiply(x=w4717, y=60.0) -> (x*y=w4724:dbl)
                n3442 = Multiply(x=1.2 ("y"), y=0.949) -> (x*y=w4693:dbl)
                n3443 = Multiply(x=1.2 ("y"), y=0.8166) -> (x*y=w4697:dbl)
                n3444 = Multiply(x=1.2 ("y"), y=0.851) -> (x*y=w4692:dbl)
                n3445 = local read "FF 2"() -> (w4716:dbl)
                n3446 = Absolute Value(x=w4724) -> (abs(x)=w4722:dbl)
                n3447 = case shown="13.." w4716 {
                  tunnel: [1 2 3] -> w4714
                  frame 0..10, Default {
                    # "Normal"
                  }
                  frame 11, 12 {
                  }
                  frame 13.. {
                  }
                }
                "FF STATE" <- w4714
                n3448 = local read "TEMP"() -> (w4677:dbl)
                n3449 = local read item#-1() -> (w4691)
                n3450 = Less?(x=w4691, y=w4697) -> (x < y?=w4694:bool)
                n3451 = In Range and Coerce(upper limit=w4693, x=w4691, lower limit=w4692) -> (In Range?=w4695:bool)  [unwired: 1 out]
                n3452 = case shown="3601.." w4722 {
                  tunnel: [1 2 3] -> w4720
                  frame 0..3000, Default {
                    # "Normal"
                  }
                  frame 3001..3600 {
                  }
                  frame 3601.. {
                  }
                }
                n3453 = case shown="11.." w4718 {
                  tunnel: [1 3] -> w4719
                  frame 1..10, Default {
                  }
                  frame 11.. {
                  }
                }
                "NL STATE" <- w4719
                n3454 = Multiply(x=1.2 ("y"), y=0.95) -> (x*y=w4707:dbl)
                n3455 = Multiply(x=w4689, y=0.954) -> (x*y=w4681:dbl)
                n3456 = Or(x=w4694, y=w4695) -> (x .or. y?=w4696:bool)
                n3457 = Greater Or Equal?(x=w4691, y=w4707) -> (x >= y?=w4704:bool)
                n3458 = Multiply(x=w4689, y=0.99) -> (x*y=w4678:dbl)
                n3459 = Greater Or Equal?(x=w4677, y=w4678) -> (x >= y?=w4683:bool)
                n3460 = Greater Or Equal?(x=w4677, y=w4681) -> (x >= y?=w4680:bool)
                n3461 = case shown="0, 1, Default" w4691 {
                  tunnel: [1 3] -> w4708
                  frame 0, 1, Default {
                  }
                  frame 2.. {
                  }
                }
                n3462 = case shown="True" w4704 {
                  tunnel: [1 3] -> w4709
                  frame False {
                  }
                  frame True {
                  }
                }
                n3463 = case shown="True" w4696 {
                  tunnel: [1 2] -> w4710
                  frame False {
                  }
                  frame True {
                  }
                }
                n3464 = case shown="..0" w4677 {
                  tunnel: [2 3 3 1] -> w4684
                  frame 61, 62 {
                  }
                  frame 63.. {
                  }
                  frame ..0 {
                  }
                  frame 10..60, Default {
                  }
                }
                n3465 = case shown="True" w4683 {
                  tunnel: [1 3] -> w4685
                  frame False {
                  }
                  frame True {
                  }
                }
                n3466 = Number To Decimal String(number=w4720) -> (decimal integer string=w4721:string)  [unwired: 1 in]
                n3467 = case shown="True" w4680 {
                  tunnel: [1 2] -> w4686
                  frame False {
                  }
                  frame True {
                  }
                }
                n3468 = Number To Decimal String(number=1) -> (decimal integer string=→"Air temp":string)  [unwired: 1 in]
                n3469 = Number To Decimal String(number=w4714) -> (decimal integer string=→"ff_st":string)  [unwired: 1 in]
                n3470 = local write "sp_st"(w4721) -> ()
                n3471 = Number To Decimal String(number=w4719) -> (decimal integer string=→"nl_st":string)  [unwired: 1 in]
                n3472 = Build Array(w4684, w4685, w4686) -> (w4687:i32[])
                n3473 = Build Array(w4708, w4709, w4710) -> (w4711:i32[])
                n3474 = Array Max & Min(array=w4687) -> (max value=w4688:i32)  [unwired: 3 out]
                n3475 = Array Max & Min(array=w4711) -> (max value=w4712:i32)  [unwired: 3 out]
                n3476 = Number To Decimal String(number=w4688) -> (decimal integer string=w4676:string)  [unwired: 1 in]
                n3477 = Number To Decimal String(number=w4712) -> (decimal integer string=→"Stroke Ln 2":string)  [unwired: 1 in]
                n3478 = local write "temp_st"(w4676) -> ()
              }
              frame True {
                w4774 = 65.0 ("y")
                # "Healthy -1\nWarning -2\nError -3"
                n3479 = local read "TEMP"() -> (w4785:dbl)
                n3480 = local read "NORMAL LOAD"() -> (w4789:dbl)
                n3481 = local read "Set Hz"() -> (w4787:dbl)
                n3482 = Multiply(x=1.2 ("y"), y=0.949) -> (x*y=w4769:dbl)
                n3483 = Multiply(x=1.2 ("y"), y=0.8166) -> (x*y=w4765:dbl)
                n3484 = Multiply(x=1.2 ("y"), y=0.851) -> (x*y=w4770:dbl)
                n3485 = Multiply(x=w4774, y=0.954) -> (x*y=w4781:dbl)
                n3486 = Multiply(x=w4774, y=0.99) -> (x*y=w4784:dbl)
                n3487 = Greater Or Equal?(x=w4785, y=w4784) -> (x >= y?=w4779:bool)
                n3488 = Multiply(x=w4787, y=60.0) -> (x*y=w4793:dbl)
                n3489 = Greater Or Equal?(x=w4785, y=w4781) -> (x >= y?=w4782:bool)
                n3490 = local read "FF 2"() -> (w4788:dbl)
                n3491 = local read item#-1() -> (w4771)
                n3492 = Less?(x=w4771, y=w4765) -> (x < y?=w4768:bool)
                n3493 = In Range and Coerce(upper limit=w4769, x=w4771, lower limit=w4770) -> (In Range?=w4767:bool)  [unwired: 1 out]
                n3494 = Absolute Value(x=w4793) -> (abs(x)=w4791:dbl)
                n3495 = case shown="63.." w4785 {
                  tunnel: [2 3 3 1] -> w4778
                  frame 61, 62 {
                  }
                  frame 63.. {
                  }
                  frame ..0 {
                  }
                  frame 10..60, Default {
                  }
                }
                n3496 = case shown="True" w4779 {
                  tunnel: [1 3] -> w4777
                  frame False {
                  }
                  frame True {
                  }
                }
                n3497 = case shown="True" w4782 {
                  tunnel: [1 2] -> w4776
                  frame False {
                  }
                  frame True {
                  }
                }
                n3498 = Multiply(x=1.2 ("y"), y=0.95) -> (x*y=w4755:dbl)
                n3499 = case shown="1..10, Default" w4789 {
                  tunnel: [1 3] -> w4796
                  frame 1..10, Default {
                  }
                  frame 11.. {
                  }
                }
                n3500 = case shown="0..10, Default" w4788 {
                  tunnel: [1 2 3] -> w4795
                  frame 0..10, Default {
                  }
                  frame 11, 12 {
                  }
                  frame 13.. {
                  }
                }
                n3501 = case shown="3601.." w4791 {
                  tunnel: [1 2 3] -> w4790
                  frame 0..3000, Default {
                    # "Normal"
                  }
                  frame 3001..3600 {
                  }
                  frame 3601.. {
                  }
                }
                n3502 = Or(x=w4768, y=w4767) -> (x .or. y?=w4766:bool)
                n3503 = Greater Or Equal?(x=w4771, y=w4755) -> (x >= y?=w4758:bool)
                n3504 = case shown="0, 1, Default" w4771 {
                  tunnel: [1 3] -> w4754
                  frame 0, 1, Default {
                  }
                  frame 2.. {
                  }
                }
                n3505 = case shown="True" w4758 {
                  tunnel: [1 3] -> w4753
                  frame False {
                  }
                  frame True {
                  }
                }
                n3506 = case shown="True" w4766 {
                  tunnel: [1 2] -> w4752
                  frame False {
                  }
                  frame True {
                  }
                }
                n3507 = Build Array(w4778, w4777, w4776) -> (w4775:i32[])
                n3508 = Number To Decimal String(number=w4790) -> (decimal integer string=→"sp_st":string)  [unwired: 1 in]
                n3509 = Array Max & Min(array=w4775) -> (max value=w4772:i32)  [unwired: 3 out]
                "TEMP STATE" <- w4772
                n3510 = Number To Decimal String(number=w4796) -> (decimal integer string=w4799:string)  [unwired: 1 in]
                n3511 = Number To Decimal String(number=w4795) -> (decimal integer string=w4797:string)  [unwired: 1 in]
                n3512 = Number To Decimal String(number=w4772) -> (decimal integer string=→"temp_st":string)  [unwired: 1 in]
                n3513 = Build Array(w4754, w4753, w4752) -> (w4751:i32[])
                n3514 = local write "nl_st"(w4799) -> ()
                n3515 = local write "ff_st"(w4797) -> ()
                n3516 = Number To Decimal String(number=1) -> (decimal integer string=w4794:string)  [unwired: 1 in]
                n3517 = Array Max & Min(array=w4751) -> (max value=w4750:i32)  [unwired: 3 out]
                n3518 = local write "Air temp"(w4794) -> ()
                n3519 = Number To Decimal String(number=w4750) -> (decimal integer string=w4749:string)  [unwired: 1 in]
                n3520 = local write "Stroke Ln 2"(w4749) -> ()
              }
            }
            n3521 = local read "Stroke Ln 2"() -> (w4661:string)
            n3522 = local read "nl_st"() -> (w4667:string)
            n3523 = local read "ff_st"() -> (w4664:string)
            n3524 = local read "sp_st"() -> (w4665:string)
            n3525 = local read "temp_st"() -> (w4666:string)
            n3526 = local read "Air temp"() -> (w4660:string)
            n3527 = Replace Array Subset(array="in", new element #1=w4667, index #1=1 ("index"), new element #2=w4664, index #2=2 ("index"), new element #3=w4666, index #3=3 ("index"), new element #4=w4665, index #4=4 ("index"), new element #5=w4661, index #5=5 ("index"), new element #6=w4660, index #6=6 ("index"), new element #7="Sensor State" ("new element/subarray"), index #7=0 ("index")) -> (→"out":string[])
          }
        }
        n3528 = Wait (ms)(milliseconds to wait=u32 10) -> ()  [unwired: 1 out]
        n3529 = local read "Quit"() -> (w4655:bool)
      }
      n3530 = while {
        stop <- w4630 stop-if-true
        n3531 = local read "run replace"() -> (w4632:bool)
        n3532 = Wait (ms)(milliseconds to wait=u32 100) -> ()  [unwired: 1 out]
        n3533 = Equal?(x="FLAG 2", y=0.0) -> (x = y?=w4633:bool)
        n3534 = case shown="True" w4633 {
          frame False {
          }
          frame True {
            n3535 = local write "FLAG 2"(100.0 ("FLAG 2")) -> ()
            n3536 = call <vilib>:"Read Characters From File.vi"("file path (dialog if empty)"=path "C:/LAB-IQ-NXT/WO 2449 TT.sig", "convert eol? (no:F)"=FALSE ("append to file? (new file:F)")) -> ("character string"=w4636:string)  [unwired: 4 in, 3 out]
            n3537 = call <vilib>:"Read Characters From File.vi"("file path (dialog if empty)"=path "C:/LAB-IQ-NXT/WO 2449 TRH.sig", "convert eol? (no:F)"=FALSE ("append to file? (new file:F)")) -> ("character string"=w4637:string)  [unwired: 4 in, 3 out]
            n3538 = Decimal String To Number(string=w4636) -> (number=w4638:i32)  [unwired: 2 in, 1 out]
            n3539 = local write "Total No. of Tests"(w4638) -> ()
            n3540 = Decimal String To Number(string=w4637) -> (number=w4641:i32)  [unwired: 2 in, 1 out]
            n3541 = local write "SEN.RUN HRS"(w4641) -> ()
          }
        }
        n3542 = case shown="True" w4632 {
          frame False {
          }
          frame True {
            n3543 = Equal?(x="FLAG 4", y=0.0) -> (x = y?=w4645:bool)
            n3544 = case shown="False" w4645 {
              frame False {
                n3545 = Get Date/Time In Seconds() -> (seconds since 1Jan1904=w4651:timestamp)
                n3546 = local read "START 3"() -> (w4649:dbl)
                n3547 = To Double Precision Float(number=w4651) -> (double precision float=w4650:dbl)
                n3548 = Subtract(x=w4650, y=w4649) -> (x-y=→"SENSOR TIME":dbl)
              }
              frame True {
                n3549 = Get Date/Time In Seconds() -> (seconds since 1Jan1904=w4653:timestamp)
                n3550 = local write "FLAG 4"(100.0 ("FLAG")) -> ()
                n3551 = To Double Precision Float(number=w4653) -> (double precision float=→"START 3":dbl)
              }
            }
          }
        }
        n3552 = local read "Quit"() -> (w4630:bool)
      }
      n3553 = while {
        shift-right: [w4430] -> _
        shift-left: _ -> [w4431]
        tunnel: [w4426] -> _
        i -> [w4426]
        stop <- w4425 stop-if-true
        n3554 = Wait (ms)(milliseconds to wait=u32 50 ("Refresh Rate (ms)")) -> ()  [unwired: 1 out]
        n3555 = local read "Json End Flg"() -> (w4427:bool)
        n3556 = Not(x="Upld AR 2") -> ()  [unwired: 1 out]
        n3557 = local read "Upld AR 2"() -> (w4428:bool)
        n3558 = call "Elapsed Time9"("Time Target (s)"="Sen.Upload Rate (s)", "Reset"=FALSE, "Auto Reset"=TRUE) -> ("Time has Elapsed"=w4437:bool)  [unwired: 9 in, 7 out]
        n3559 = Or(x=w4437, y=w4427) -> (x .or. y?=w4433:bool)
        n3560 = case shown="True" w4433 {
          frame False {
          }
          frame True {
            w4529 = "\"SensorName\":\"" ("string")
            w4499 = " \"},{"
            w4524 = "\",\"SensorState\":\""
            w4526 = "\",\"SensorModelNumber\":\"" ("string")
            w4525 = "\",\"SensorRuntimeHours\":\"" ("string")
            n3561 = local read "model num"() -> (w4523:string[])
            n3562 = local read "Sensor name"() -> (w4542:string[])
            n3563 = local read "run"() -> (w4513:string[])
            n3564 = local read "SENSOR TIME"() -> (w4469:dbl)
            n3565 = local read "out"() -> (w4462:string[])
            n3566 = local read "Total No. of Tests"() -> (w4467:dbl)
            n3567 = Select(t=60.0, s="Run test 3", f=3600.0) -> (s? t:f=w4477:dbl)
            n3568 = Index Array(array=w4523, index #1=1 ("index")) -> (element #1=w4522:string, element #2=w4521:string, element #3=w4520:string, element #4=w4519:string, element #5=w4518:string, element #6=w4517:string)  [unwired: 5 in]
            n3569 = Index Array(array=w4513, index #1=1 ("index")) -> (element #1=w4512:string, element #2=w4511:string, element #3=w4510:string, element #4=w4509:string, element #5=w4508:string, element #6=w4507:string)  [unwired: 5 in]
            n3570 = Index Array(array=w4542, index #1=1 ("index")) -> (element #1=w4541:string, element #2=w4540:string, element #3=w4539:string, element #4=w4538:string, element #5=w4528:string, element #6=w4527:string)  [unwired: 5 in]
            n3571 = Index Array(array=w4462, index #1=1 ("index")) -> (element #1=w4494:string, element #2=w4493:string, element #3=w4492:string, element #4=w4491:string, element #5=w4490:string, element #6=w4489:string)  [unwired: 5 in]
            n3572 = local read "SEN.RUN HRS"() -> (w4465:dbl)
            n3573 = Divide(x=w4469, y=w4477) -> (x/y=w4476:dbl)
            n3574 = Increment(x=w4476) -> (x+1=w4472:dbl)
            n3575 = Number To Decimal String(number=w4472) -> (decimal integer string=→"run hrs":string)  [unwired: 1 in]
            n3576 = Divide(x=w4465, y=3600.0 ("f")) -> (x/y=w4460:dbl)
            n3577 = Round To Nearest(number=w4460) -> (nearest integer value=w4458:dbl)
            n3578 = Number To Decimal String(number=w4458) -> (decimal integer string=w4459:string)  [unwired: 1 in]
            n3579 = Number To Decimal String(number=w4467) -> (decimal integer string=w4468:string)  [unwired: 1 in]
            n3580 = local read "Model No"() -> (w4473:string)
            n3581 = local read "UUID"() -> (w4568:string)
            n3582 = local read "Serial No"() -> (w4572:string)
            n3583 = local read "Secret Key"() -> (w4573:string)
            n3584 = Concatenate Strings("\",\"MachineSerialNumber\":\"" ("string"), w4572) -> (w4576:string)
            n3585 = Concatenate Strings("\",\"ModelNumber\":\"" ("string"), w4473) -> (w4474:string)
            n3586 = Concatenate Strings("\",\"MachineRuntimeHours\":\"" ("string"), w4459) -> (w4577:string)
            n3587 = Concatenate Strings("\",\"MachineRuntimeCycles\":\"", w4468) -> (w4570:string)
            n3588 = Concatenate Strings(w4526, w4522) -> (w4556:string)
            n3589 = Concatenate Strings(w4525, w4512) -> (w4557:string)
